vi "current_path.vi"() -> (0 "name":string, 1 "stripped path":path)   [LabVIEW 2018]
doc: "This subVI returns the name and the stripped path of the calling VI. This is different from the shipping Current Path.vi in that the LabVIEW one returns something different if it is part of a .vi file or is inside a .llb file or is an executable file. The subVI in this .llb file gives you the directory of execution of the VI running it and it is always the same, the correct one."
panel:
  # "This VI returns the name of the VI and the stripped path of the file. This is different from the \nLabVIEW Current VI's Path constant. The constant returns a different path if it is part of a .vi \nfile, inside an .llb, or if it is an executable file. This VI returns the path of the running VI, even if\nit is part of a .vi file, inside an .llb, or if it is an executable file."
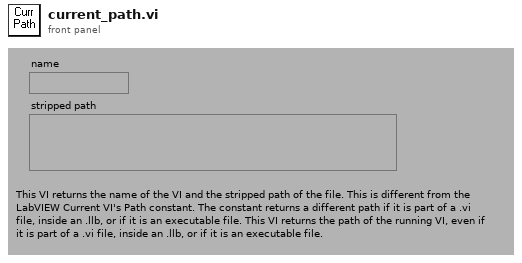
[diagram p1: front panel]
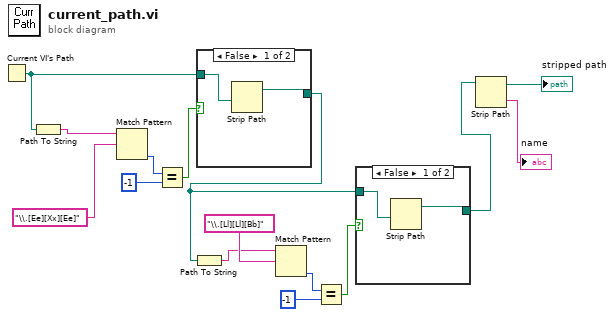
[diagram p0: block diagram]
diagram:
  n1 = Current VI's Path() -> (path=w10:path)
  n2 = Path To String(path=w10) -> (string=w11:string)
  n3 = Match Pattern(string=w11, regular expression="\\.[Ee][Xx][Ee]") -> (offset past match=w14:i32)  [unwired: 1 in, 3 out]
  n4 = Equal?(x=w14, y=-1) -> (x = y?=w12:bool)
  n5 = case shown="False" w12 {
    tunnel: [w17 w18] -> w2
    tunnel: w10 -> [w16 w18]
    frame False {
      n6 = Strip Path(path=w16) -> (stripped path=w17:path)  [unwired: 1 out]
    }
    frame True {
    }
  }
  n7 = Path To String(path=w2) -> (string=w6:string)
  n8 = Match Pattern(string=w6, regular expression="\\.[Ll][Ll][Bb]") -> (offset past match=w3:i32)  [unwired: 1 in, 3 out]
  n9 = Equal?(x=w3, y=-1) -> (x = y?=w5:bool)
  n10 = case shown="False" w5 {
    tunnel: [w20 w21] -> w1
    tunnel: w2 -> [w19 w21]
    frame False {
      n11 = Strip Path(path=w19) -> (stripped path=w20:path)  [unwired: 1 out]
    }
    frame True {
    }
  }
  n12 = Strip Path(path=w1) -> (stripped path=→"stripped path":path, name=→"name":string)
